vi "Reading from Hardware - STR to DBL.vi"() -> ()   [LabVIEW 2015]
panel:
  out "Voltage Reading":dbl
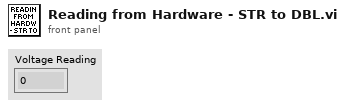
[diagram p1: front panel]
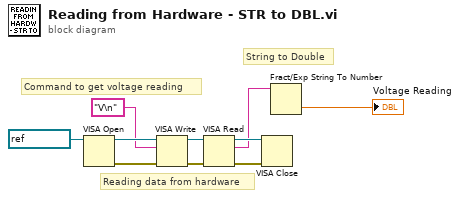
[diagram p0: block diagram]
diagram:
  # "String to Double"
  # "Reading data from hardware"
  # "Command to get voltage reading"
  n1 = VISA Open(VISA resource name=refnum<visa-resource-name> "COM3") -> (VISA resource name=w10:refnum<visa-resource-name>, error out=w9:errorcluster)  [unwired: 4 in]
  n2 = VISA Write(VISA resource name=w10, write buffer="V\n", error in (no error)=w9) -> (VISA resource name out=w8:refnum<visa-resource-name>, error out=w7:errorcluster)  [unwired: 1 out]
  n3 = VISA Read(VISA resource name=w8, error in (no error)=w7) -> (VISA resource name out=w6:refnum<visa-resource-name>, read buffer=w2:string, error out=w5:errorcluster)  [unwired: 1 in, 1 out]
  n4 = VISA Close(VISA resource name=w6, error in (no error)=w5) -> ()  [unwired: 1 out]
  n5 = Fract/Exp String To Number(string=w2) -> (number=→"Voltage Reading":dbl)  [unwired: 3 in, 1 out]
